vi "Calc Elements to Read.vi"(9 "Sync Guard Data Length":u32, 10 "Elements in FIFO":u32, 11 "Data Size":u32) -> (2 "# Data Sets To Read":u32, 3 "# Elements to Read":u32)   [LabVIEW 2023]
doc: "Author: Scott Hannahs <sth@magnet.fsu.edu>\nCopyright 2018 Florida State University, All rights reserved."
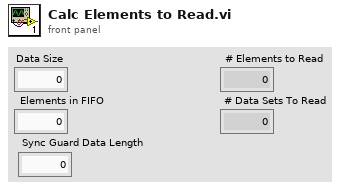
[diagram p1: front panel]
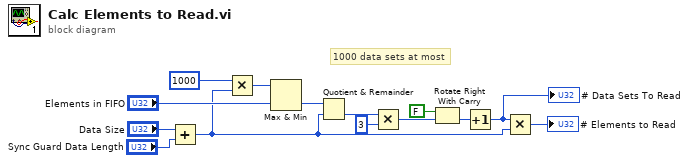
[diagram p0: block diagram]
diagram:
  # "1000 data sets at most"
  n1 = Add(x="Data Size", y="Sync Guard Data Length") -> (x+y=w2:u32)
  n2 = Multiply(x=u32 1000, y=w2) -> (x*y=w3:u32)
  n3 = Max & Min(x=w3, y="Elements in FIFO") -> (min(x,y)=w5:u32)  [unwired: 1 out]
  n4 = Quotient & Remainder(x=w5, y=w2) -> (floor(x/y)=w7:u32)  [unwired: 1 out]
  n5 = Multiply(x=w7, y=u32 3) -> (x*y=w8:u32)
  n6 = Rotate Right With Carry(2:w8, 3:FALSE ("carry")) -> (0:w10:u32)  [unwired: 1 out]
  n7 = Increment(x=w10) -> (x+1=w14:u32)
  "# Data Sets To Read" <- w14
  n8 = Multiply(x=w14, y=w2) -> (x*y=→"# Elements to Read":u32)
